vi "NumToDigits(I8).vi"(8 "error in (no error)":errorcluster caption="错误输入（无错误）", 10 "基数 (10)":i8=10, 11 "输入数值":i8) -> (0 "error out":errorcluster caption="错误输出", 2 "总位数":i32, 3 "位数数组":i8[](array[numeric]))   [LabVIEW 2012]
doc: "Converts a single I32 into an array of digits, in order of increasing significance. If the input number is negative, the most significant digit (last element of the array) is also negative. All other digits are always non-negative. By default, the output digits are the digits used to represent the number in base 10, though the base can be changed. For example, the binary representation can be obtained by wiring the value 2 to the Base input. Note that Base is coerced to a minimum value of 2.\n\nAs long as no coersion is required, the original number can be recreated as\nN = Digits[0] * Base^0 + Digits[1] * Base^1 + Digits[2] * Base^2 + ... + Digits[n] * Base^n\n\nFreeware from Moore Good Ideas, www.mooregoodideas.com. Do not remove this line."
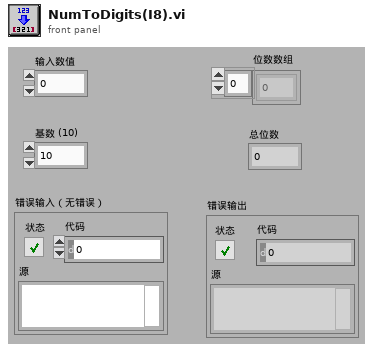
[diagram p1: front panel]
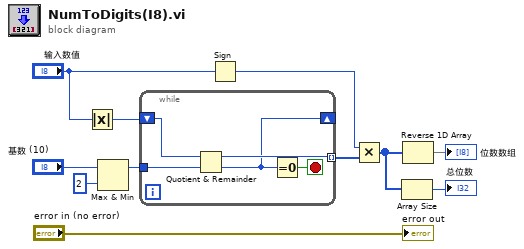
[diagram p0: block diagram]
diagram:
  n1 = Absolute Value(x="输入数值") -> (abs(x)=w3:i8)
  n2 = Max & Min(x="基数 (10)", y=i8 2) -> (max(x,y)=w10:i8)  [unwired: 1 out]
  n3 = while {
    tunnel: w10 -> [w16]
    tunnel: [w14] -> w7 mode=indexing
    shift-right: [w12] -> _
    shift-left: w3 -> [w13]
    stop <- w15 stop-if-true
    n4 = Quotient & Remainder(x=w13, y=w16) -> (x-y*floor(x/y)=w14:i8, floor(x/y)=w12:i8)
    n5 = Equal To 0?(x=w12) -> (x = 0?=w15:bool)
  }
  n6 = Sign(1:"输入数值") -> (0:w6:i8)
  n7 = Multiply(x=w6, y=w7) -> (x*y=w5:i8[])
  n8 = Array Size(array=w5) -> (size(s)=→"总位数":i32)
  n9 = Reverse 1D Array(array=w5) -> (reversed array=→"位数数组":i8[])
  "error out" <- "error in (no error)"
